vi "Write.vi"(8 "error in (no error)":errorcluster, 10 "element":variant, 11 "NetworkStreamWriter in":refnum<class "NetworkStreamWriter.lvclass">) -> (0 "error out":errorcluster, 3 "NetworkStreamWriter out":refnum<class "NetworkStreamWriter.lvclass">)   [LabVIEW 2011, in "NetworkStreamWriter.lvclass"]
doc: "Returns the requested value (either the next element available in the buffer or the most recent element). If there are no elements available in the queue, this VI will return the last valid value it returned.\n\nWrites the requested value to the internal queue, which will be sent across the network asynchronously by the WriterDaemon."
uses:
  NetworkStreamWriter.lvclass
  Shared/message.ctl
  NetworkStreamWriter.lvclass/NetworkStreamWriter.ctl
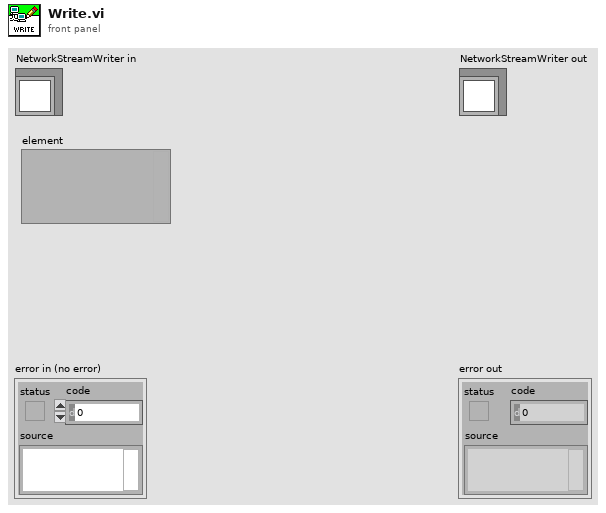
[diagram p1: front panel]
types:
  T1 = typedef "message.ctl" = cluster{"Data":variant, "Time since start (s)":dbl}
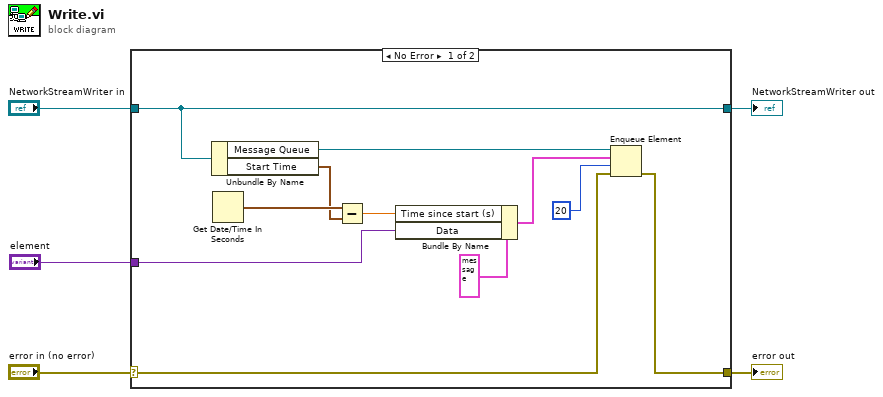
[diagram p0: block diagram]
diagram:
  n1 = case shown="No Error" "error in (no error)" {
    selector: "error in (no error)" -> [w14 w18]
    tunnel: [w12 w18] -> w4
    tunnel: [w16 w17] -> w2
    tunnel: "NetworkStreamWriter in" -> [w16 w17]
    tunnel: "element" -> [w7 _]
    frame No Error {
      n2 = Unbundle By Name(w16) -> ("Message Queue"=w15:refnum<queue>, "Start Time"=w10:timestamp)
      n3 = Get Date/Time In Seconds() -> (seconds since 1Jan1904=w11:timestamp)
      n4 = Subtract(x=w11, y=w10) -> (x-y=w8:dbl)
      n5 = Bundle By Name(cluster=T1 {"Data"=variant, "Time since start (s)"=0.0} ("Message"), "Time since start (s)"=w8, "Data"=w7) -> (w6:T1)
      n6 = Enqueue Element(queue=w15, element=w6, timeout in ms (-1)=20, error in (no error)=w14) -> (error out=w12:errorcluster)  [unwired: 2 out]
    }
    frame Error {
    }
  }
  "error out" <- w4
  "NetworkStreamWriter out" <- w2
